vi "Main.vi"(10 "Module Admin":refnum<class "Delacor_lib_QMH_Module Admin.lvclass">, 11 "Sequence Context In":refnum<k7>) -> ()   [LabVIEW 2015, in "TestStand Manager_DQMH.lvlib"]
doc: "This application is based on the Delacor QMH project template. This particular module is headless, it has no UI, which is why the Show Panel, Hide Panel, and related events are unused.\n\nThe purpose of the TestStand Manager_DQMH Module is to check if the TestStand sequence is terminated. If so, it sends the request to stop all Thermal Chamber DQMH modules. This Module is only used when running the TestStand Examples.\n\n_____\nBased on Delacor QMH Project Template 2.0.0.62.\nReviewed and updated to match QMH Project Template 4.0.\n\n<b>Note:</b> This VI was modified by the <b>Validate DQMH Module</b> tool to upgrade it to the DQMH 2.1 approach to stopping a singleton module.\n\n<b>Note:</b> This VI was modified by the <b>Validate DQMH Module</b> tool to upgrade it to the DQMH 3.0 implementation of the 'Show Diagram' message, which checks the password-protected status of the Main VI before showing the diagram.\n____\nDelacor QMH Thermal Chamber Examples 4.0.0.21\nCopyright (c) 2018, Delacor"
uses:
  TestStand Manager_DQMH.lvlib
  Module Data--cluster.ctl
  <vilib>/Delacor/Delacor QMH/Libraries/Message Queue_class/Delacor_lib_QMH_Message Queue.lvclass
  <vilib>/Delacor/Delacor QMH/Libraries/Message Queue_class/Delacor_lib_QMH_Enqueue Message (Single).vi
  <vilib>/ErrorRing/Error Ring.xnode
  <vilib>/Utility/error.llb/Error Cluster From Error Code.vi
  <vilib>/Delacor/Delacor QMH/Libraries/Module Admin_class/Delacor_lib_QMH_Module Admin.lvclass
  Stop Argument--cluster.ctl
  <vilib>/addons/TestStand/_TSUtility.llb/TestStand - Status Monitor.ctl
  Thermal Chamber Controller_DQMH/Thermal Chamber Controller_DQMH.lvlib
  Device Under Test_Cloneable_DQMH/Device Under Test_Cloneable_DQMH.lvlib
panel:
  out "error out":errorcluster
  out "Status":string
  # "The purpose of the TestStand Manager_DQMH Module is to check if the TestStand sequence is terminated. If so, it sends the request to stop all Thermal Chamber DQMH modules. This Module is only used when running the TestStand Examples."
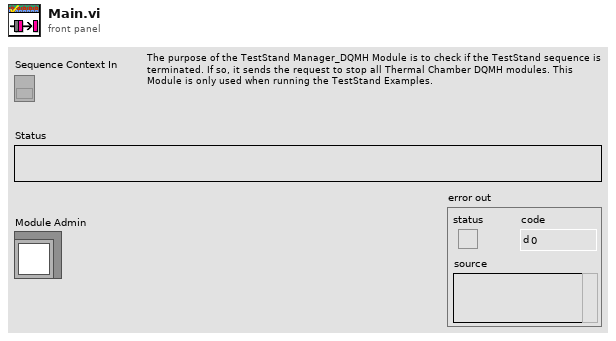
[diagram p1: front panel]
types:
  T1 = typedef "TestStand Manager_DQMH.lvlib/Request Events--cluster.ctl" = cluster{"Stop Module":refnum<user-event>, "Show Panel":refnum<user-event>, "Hide Panel":refnum<user-event>, "Get Module Execution Status":refnum<user-event>, "Show Diagram":refnum<user-event>}
  T2 = typedef "TestStand Manager_DQMH.lvlib/Module Data--cluster.ctl" = cluster{"Status":string, "Status Monitor":T3}
  T3 = typedef "TestStand - Status Monitor.ctl" = cluster{"Sequence Context":refnum<k7>, "Execution":refnum<k7>, "Termination Monitor":refnum<k7>}
  T4 = typedef "TestStand Manager_DQMH.lvlib/Stop Argument--cluster.ctl" = cluster{"Origin":string, "Exit via Stop Module Req?":bool, "Wait for Module to stop?":bool}
  T5 = enum32{"invalid lock state", "Not Locked", "Locked (No Password)", "Password-protected"}
  T6 = enum32{"Invalid", "Standard", "Closed", "Hidden", "Minimized", "Maximized"}
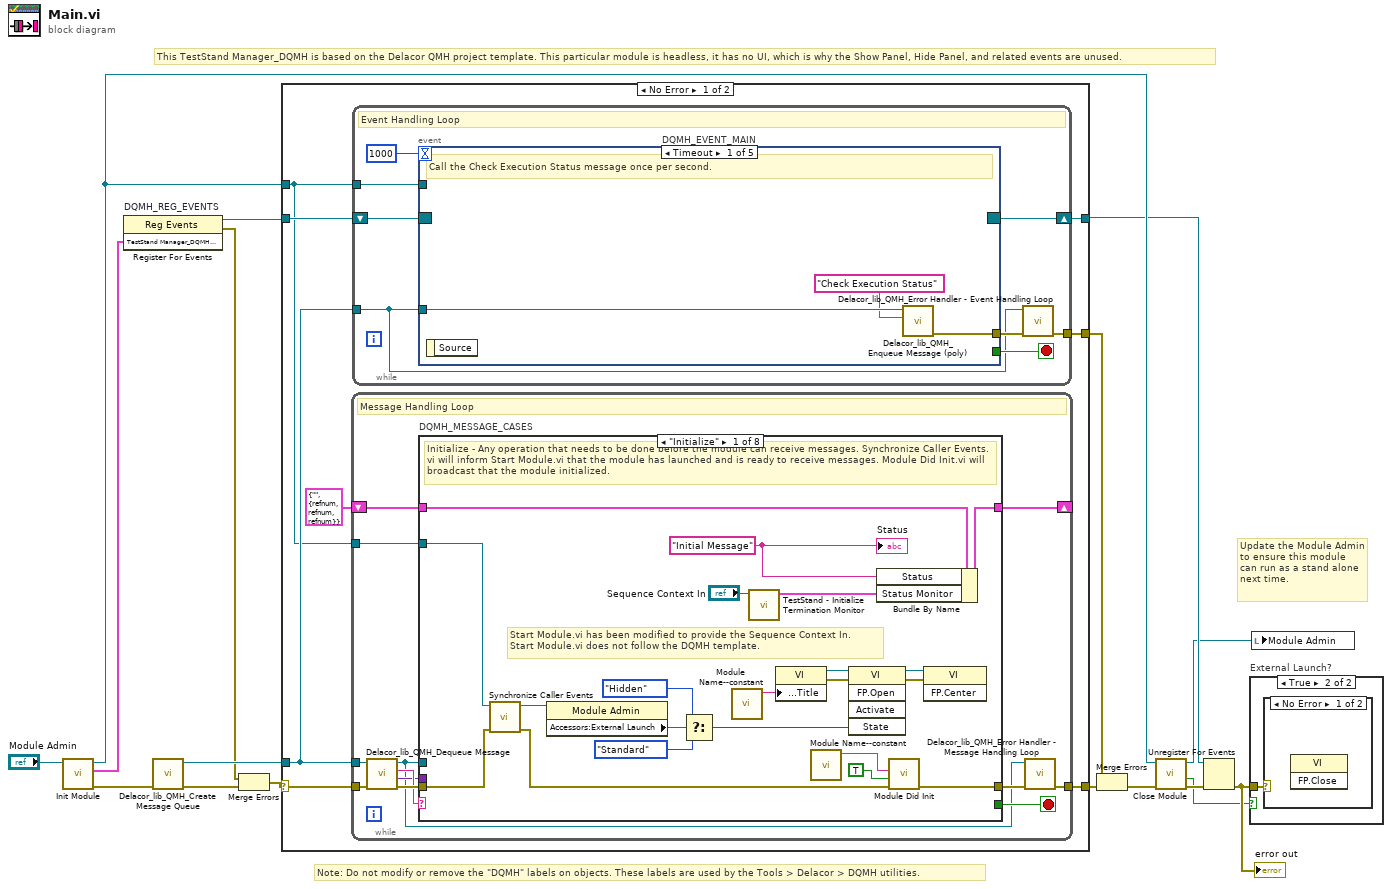
[diagram p0: block diagram]
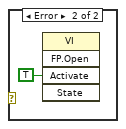
[diagram p3: hidden frame]
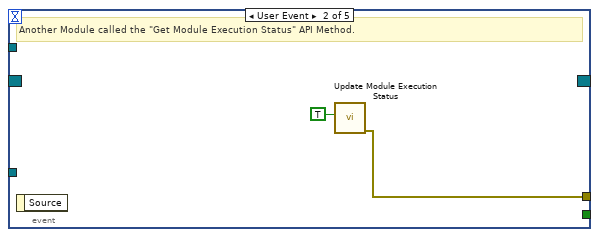
[diagram p4: hidden frame]
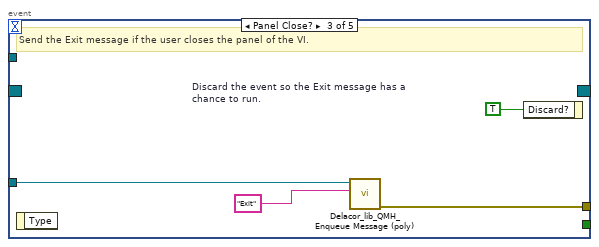
[diagram p5: hidden frame]
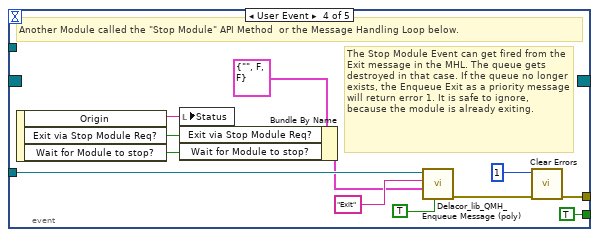
[diagram p6: hidden frame]
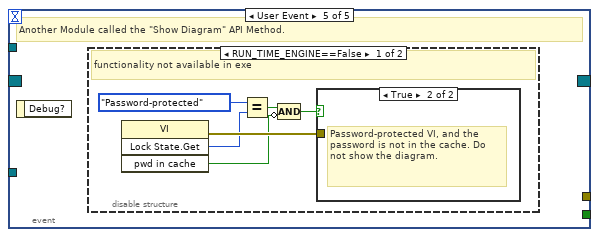
[diagram p7: hidden frame]
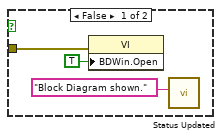
[diagram p8: hidden frame]
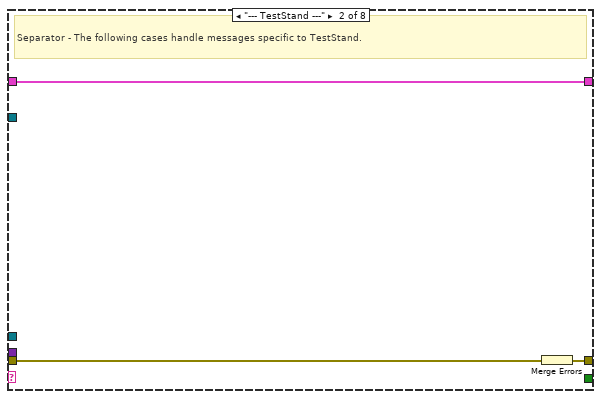
[diagram p10: hidden frame]
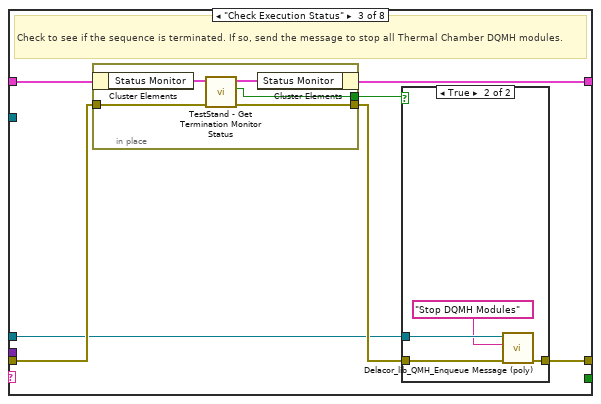
[diagram p11: hidden frame]
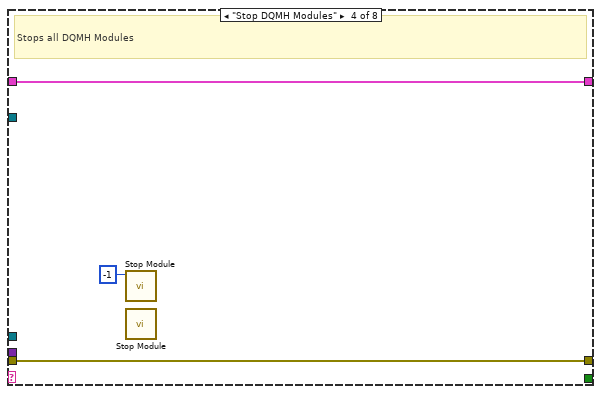
[diagram p13: hidden frame]
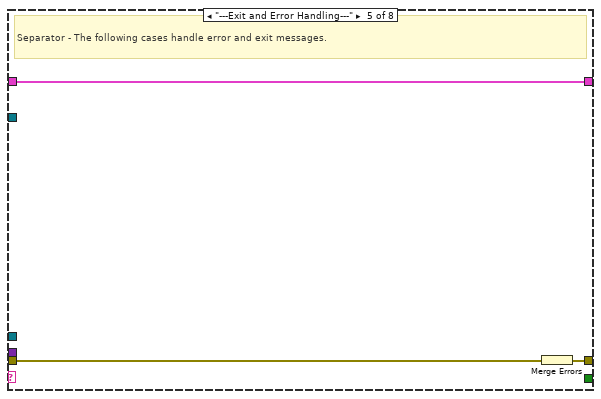
[diagram p14: hidden frame]
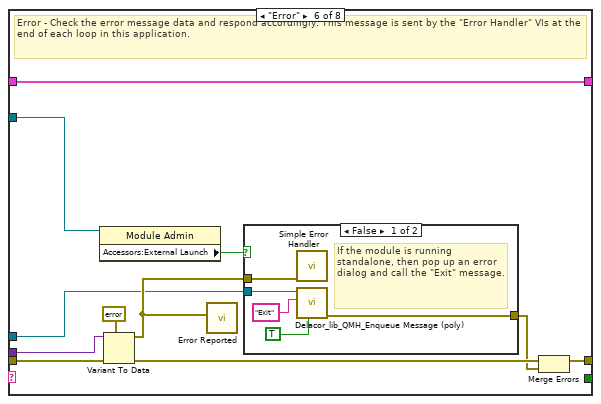
[diagram p15: hidden frame]
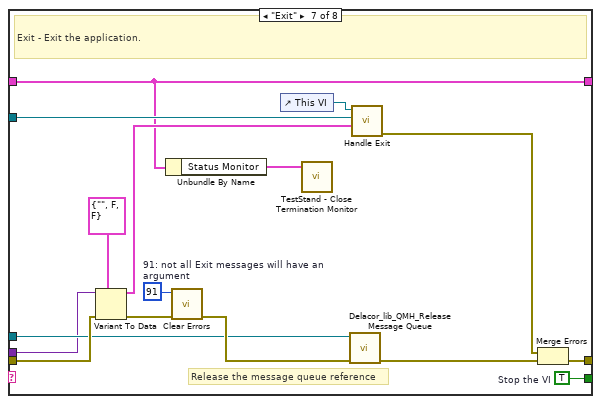
[diagram p17: hidden frame]
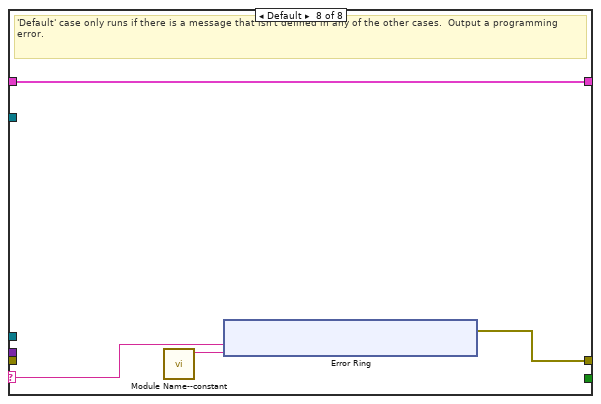
[diagram p18: hidden frame]
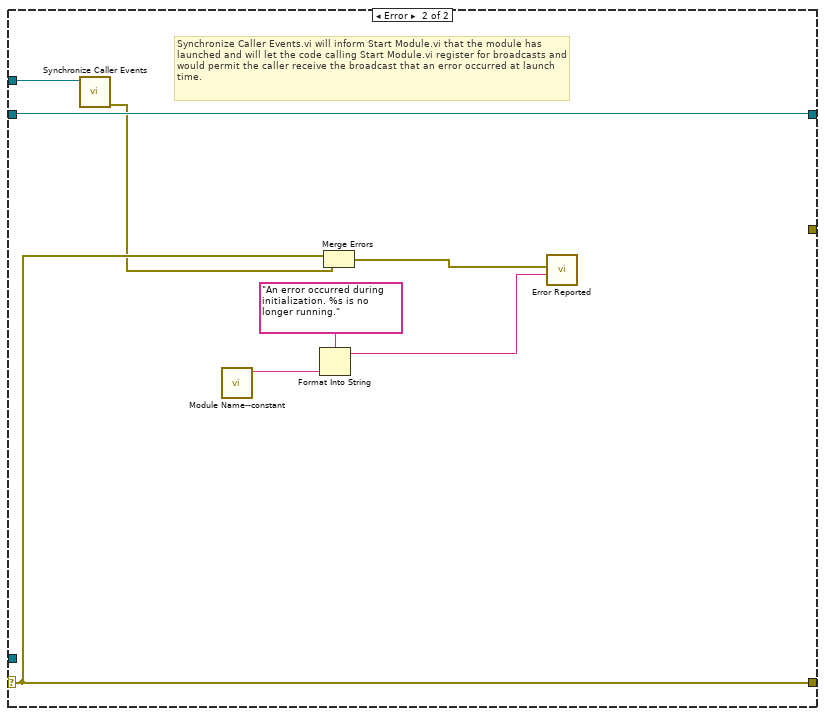
[diagram p19: hidden frame]
diagram:
  # "This TestStand Manager_DQMH is based on the Delacor QMH project template. This particular module is headless, it has no UI, which is why the Show Panel, Hide Panel, and related events are unused."
  # "Note: Do not modify or remove the \"DQMH\" labels on objects. These labels are used by the Tools > Delacor > DQMH utilities."
  # "Update the Module Admin to ensure this module can run as a stand alone next time."
  n1 = call "Init Module.vi"("Singleton Module Admin in"="Module Admin") -> ("error out"=w15:errorcluster, "TestStand Manager_DQMH Request Events"=w12:T1, "Singleton Module Admin out"=w17:refnum<class "Delacor_lib_QMH_Module Admin.lvclass">)  [unwired: 8 in]
  n2 = register-events "DQMH_REG_EVENTS"(w12) -> (reference out=w13:refnum<event-registration>, error out=w1:errorcluster)  [unwired: 2 in]
  n3 = call <vilib>:"Delacor_lib_QMH_Create Message Queue.vi"("error in (no error)"=w15) -> ("error out"=w3:errorcluster, "Message Queue out"=w11:refnum<class "Delacor_lib_QMH_Message Queue.lvclass">)  [unwired: 9 in]
  n4 = Merge Errors(w1, w3) -> (w2:errorcluster)
  n5 = case shown="No Error" w2 {
    selector: w2 -> [w19 w169]
    tunnel: [w25 w169] -> w16
    tunnel: [w24 w174] -> w14
    tunnel: w13 -> [w22 w174]
    tunnel: w11 -> [w21 _]
    tunnel: [w20 _] -> w7
    tunnel: w17 -> [w18 w170]
    frame No Error {
      n6 = while {
        tunnel: w21 -> [w67]
        shift-right: [w73] -> _
        shift-left: T2 {"Status"="", "Status Monitor"={"Sequence Context"=refnum, "Execution"=refnum, "Termination Monitor"=refnum}} ("Data Cluster") -> [w74]
        tunnel: w19 -> [w71]
        tunnel: [w65] -> w25
        tunnel: w18 -> [w64]
        stop <- w72 stop-if-true
        # "Message Handling Loop"
        n7 = call-dynamic "Delacor_lib_QMH_Dequeue Message.vi"("error in (no error)"=w71, "Message Queue in"=w67) -> ("error out"=w70:errorcluster, "Message Data"=w68:variant, "Message"=w69:string, "Message Queue out"=w66:refnum<class "Delacor_lib_QMH_Message Queue.lvclass">)  [unwired: 6 in]
        n8 = case "DQMH_MESSAGE_CASES" shown="\"Initialize\"" w69 {
          selector: w69 -> [_ _ _ _ _ _ _ w156]
          tunnel: w66 -> [_ _ w100 _ _ w125 w152 _]
          tunnel: w70 -> [w86 w99 w102 w117 w122 w132 w154 _]
          tunnel: [w80 w97 w101 w117 w120 w126 w149 w157] -> w75
          tunnel: w74 -> [w85 w98 w104 w119 w121 w131 w140 w158]
          tunnel: [w84 w98 w103 w119 w121 w131 w140 w158] -> w73
          tunnel: [_ _ _ _ _ _ w151 _] -> w72
          tunnel: w68 -> [_ _ _ _ _ w130 w148 _]
          tunnel: w64 -> [w87 _ _ _ _ w124 w141 _]
          frame "Initialize" {
            w76 = "Initial Message" ("Initial Message")
            # "Start Module.vi has been modified to provide the Sequence Context In.\nStart Module.vi does not follow the DQMH template."
            # "Initialize - Any operation that needs to be done before the module can receive messages. Synchronize Caller Events.vi will inform Start Module.vi that the module has launched and is ready to receive messages. Module Did Init.vi will broadcast that the module initialized."
            n9 = call "Synchronize Caller Events.vi"("error in (no error)"=w86, "Singleton Module Admin in"=w87) -> ("error out"=w81:errorcluster, "Singleton Module Admin out"=w79:refnum<class "Delacor_lib_QMH_Module Admin.lvclass">)  [unwired: 8 in]
            n10 = property on="Property Node" class="Module Admin"(reference=w79) -> ("Accessors:External Launch"=w91:bool)  [unwired: 1 in, 2 out]
            n11 = Select(t=T6."Hidden" ("State"), s=w91, f=T6."Standard" ("State")) -> (s? t:f=w88:T6)
            n12 = call "Module Name--constant.vi"() -> ("Module Name"=w96:string)  [unwired: 11 in]
            n13 = call <vilib>:"TestStand - Initialize Termination Monitor.vi"("Sequence Context In"="Sequence Context In") -> ("Status Monitor Out"=w77:T3)  [unwired: 9 in, 1 out]
            n14 = property on="Property Node" class="VI"("Front Panel.Title"=w96) -> (reference out=w94:refnum<vi>, error out=w95:errorcluster)  [unwired: 2 in]
            n15 = call "Module Name--constant.vi"() -> ("Module Name"=w82:string)  [unwired: 11 in]
            n16 = invoke on="Invoke Node" class="VI" method="FP.Open"(reference=w94, error in=w95, "State"=w88) -> (reference out=w93:refnum<vi>, error out=w92:errorcluster)  [unwired: 2 in, 3 out]
            n17 = Bundle By Name(cluster=w85, "Status"=w76, "Status Monitor"=w77) -> (w84:T2)
            n18 = call "Module Did Init.vi"("error in (no error)"=w81, "Initialized?"=TRUE, "Origin"=w82) -> ("error out"=w80:errorcluster)  [unwired: 8 in]
            n19 = invoke on="Invoke Node" class="VI" method="FP.Center"(reference=w93, error in=w92) -> ()  [unwired: 1 in, 3 out]
            "Status" <- w76
          }
          frame "--- TestStand ---" {
            # "Separator - The following cases handle messages specific to TestStand."
            n20 = Merge Errors(w99) -> (w97:errorcluster)
          }
          frame "Check Execution Status" {
            # "Check to see if the sequence is terminated. If so, send the message to stop all Thermal Chamber DQMH modules."
            n21 = in-place {
              in-place-border: w102 -> [w111]
              in-place-border: [w110] -> w106
              in-place-border: [w109] -> w105
              n22 = in-place-cluster #1(w104) -> ("Status Monitor"=w108:T3)
              n23 = call <vilib>:"TestStand - Get Termination Monitor Status.vi"("error in (no error)"=w111, "Status Monitor In"=w108) -> ("error out"=w110:errorcluster, "Terminating or Aborting"=w109:bool, "Status Monitor Out"=w107:T3)  [unwired: 7 in]
              n24 = in-place-cluster #1("Status Monitor"=w107) -> (w103:T2)
            }
            n25 = case shown="True" w105 {
              tunnel: w106 -> [w112 w116]
              tunnel: [w112 w115] -> w101
              tunnel: w100 -> [_ w114]
              frame False {
              }
              frame True {
                n26 = call-poly <vilib>:"Delacor_lib_QMH_Enqueue Message (poly).vi"("error in (no error)"=w116, "Message"="Stop DQMH Modules", "Message Queue in"=w114) -> ("error out"=w115:errorcluster)  [unwired: 7 in, 1 out]
              }
            }
          }
          frame "Stop DQMH Modules" {
            # "Stops all DQMH Modules"
            n27 = call "Stop Module.vi"("Module ID"=-1) -> ()  [unwired: 10 in, 1 out]
            n28 = call "Stop Module.vi"() -> ()  [unwired: 11 in, 1 out]
          }
          frame "---Exit and Error Handling---" {
            # "Separator - The following cases handle error and exit messages."
            n29 = Merge Errors(w122) -> (w120:errorcluster)
          }
          frame "Error" {
            # "Error - Check the error message data and respond accordingly. This message is sent by the \"Error Handler\" VIs at the end of each loop in this application."
            n30 = property on="Property Node" class="Module Admin"(reference=w124) -> ("Accessors:External Launch"=w123:bool)  [unwired: 1 in, 2 out]
            n31 = Variant To Data(error in=w132, type=errorcluster {"status"=FALSE, "code"=0, "source"=""} ("error constant"), Variant=w130) -> (data=w133:errorcluster, error out=w128:errorcluster)
            n32 = call "Error Reported.vi"("Error"=w133) -> ()  [unwired: 10 in, 1 out]
            n33 = case shown="False" w123 {
              tunnel: [w138 _] -> w127
              tunnel: w125 -> [w137 _]
              tunnel: w133 -> [w134 _]
              frame False {
                # "If the module is running standalone, then pop up an error dialog and call the \"Exit\" message."
                n34 = call <vilib>:"Simple Error Handler.vi"("error in (no error)"=w134) -> ()  [unwired: 4 in, 5 out]
                n35 = call-poly <vilib>:"Delacor_lib_QMH_Enqueue Message (poly).vi"("Priority Message? (F)"=TRUE, "Message"="Exit", "Message Queue in"=w137) -> ("error out"=w138:errorcluster)  [unwired: 7 in, 1 out]
              }
              frame True {
                # "If the module was launched externally, calling the Error Reported broadcast VI is the only action performed by the \"Error\" message. The module's caller can then process the error appropriately."
              }
            }
            n36 = Merge Errors(w128, w127) -> (w126:errorcluster)
          }
          frame "Exit" {
            w146 = 91  # 91: not all Exit messages will have an argument
            w151 = TRUE  # Stop the VI
            # "Release the message queue reference"
            # "Exit - Exit the application."
            n37 = Variant To Data(error in=w154, type=T4 {"Origin"="", "Exit via Stop Module Req?"=FALSE, "Wait for Module to stop?"=FALSE} ("Stop Argument"), Variant=w148) -> (data=w144:T4, error out=w147:errorcluster)
            n38 = Unbundle By Name(w140) -> ("Status Monitor"=w139:T3)
            n39 = call <vilib>:"Clear Errors.vi"("error in (no error)"=w147, "specific error code to clear (0: all)"=w146) -> ("error out"=w153:errorcluster)  [unwired: 4 in, 1 out]
            n40 = control-ref of="This VI"() -> (w142:refnum<vi>)
            n41 = call <vilib>:"TestStand - Close Termination Monitor.vi"("Status Monitor In"=w139) -> ()  [unwired: 10 in, 1 out]
            n42 = call-dynamic "Delacor_lib_QMH_Release Message Queue.vi"("error in (no error)"=w153, "Message Queue"=w152) -> ("error out"=w150:errorcluster)  [unwired: 9 in]
            n43 = call "Handle Exit.vi"("Stop Argument"=w144, "Admin in"=w141, "VI reference"=w142) -> ("error out"=w143:errorcluster)  [unwired: 7 in, 1 out]
            n44 = Merge Errors(w143, w150) -> (w149:errorcluster)
          }
          frame Default {
            # "'Default' case only runs if there is a message that isn't defined in any of the other cases.  Output a programming error."
            n45 = call "Module Name--constant.vi"() -> ("Module Name"=w155:string)  [unwired: 11 in]
            n46 = xnode "Error Ring"("parameter 0"=w156, "parameter 1"=w155) -> ("error out"=w157:errorcluster)
          }
        }
        n47 = call-dynamic "Delacor_lib_QMH_Error Handler - Message Handling Loop.vi"("error in (no error)"=w75, "Message Queue in"=w66) -> ("dup error in"=w65:errorcluster)  [unwired: 8 in, 1 out]
      }
      n48 = while {
        tunnel: w21 -> [w26]
        shift-right: [w32] -> w24
        shift-left: w22 -> [w33]
        tunnel: [w29] -> w20
        tunnel: w18 -> [w28]
        stop <- w30 stop-if-true
        # "Event Handling Loop"
        n49 = event "DQMH_EVENT_MAIN" shown="[0] Timeout" {
          selector: w33 -> [_ _ _ _ _]
          dyn-events: [_ _ _ _ _] -> w32
          timeout: 1000 -> [_ _ _ _ _]
          tunnel: [_ _ _ TRUE ("Discard?") _] -> w30
          tunnel: w26 -> [w36 _ w41 w52 _]
          tunnel: [w35 w38 w40 w47 _] -> w31
          tunnel: w28 -> [_ _ _ _ _]
          event Timeout {
            # "Call the Check Execution Status message once per second."
            n50 = event-data() -> ()  [unwired: 1 in, 1 out]
            n51 = call-poly <vilib>:"Delacor_lib_QMH_Enqueue Message (poly).vi"("Message"="Check Execution Status", "Message Queue in"=w36) -> ("error out"=w35:errorcluster)  [unwired: 8 in, 1 out]
          }
          event User Event {
            # "Another Module called the \"Get Module Execution Status\" API Method."
            n52 = event-data() -> ()  [unwired: 1 in, 1 out]
            n53 = call "Update Module Execution Status.vi"("Running?"=TRUE) -> ("error out"=w38:errorcluster)  [unwired: 10 in]
          }
          event Panel Close? {
            w42 = TRUE  # Discard the event so the Exit message has a chance to run.
            # "Send the Exit message if the user closes the panel of the VI."
            n54 = event-data() -> ()  [unwired: 1 in, 1 out]
            n55 = call-poly <vilib>:"Delacor_lib_QMH_Enqueue Message (poly).vi"("Message"="Exit", "Message Queue in"=w41) -> ("error out"=w40:errorcluster)  [unwired: 8 in, 1 out]
            n56 = event-data ("Event Filter Node")("Discard?"=w42) -> ()  [unwired: 1 in, 1 out]
          }
          event User Event {
            # "The Stop Module Event can get fired from the Exit message in the MHL. The queue gets destroyed in that case. If the queue no longer exists, the Enqueue Exit as a priority message will return error 1. It is safe to ignore, because the module is already exiting."
            # "Another Module called the \"Stop Module\" API Method  or the Message Handling Loop below."
            n57 = event-data() -> ("Origin"=w51:string, "Exit via Stop Module Req?"=w45:bool, "Wait for Module to stop?"=w44:bool)  [unwired: 1 in]
            n58 = local write "Status"(w51) -> ()
            n59 = Bundle By Name(cluster=T4 {"Origin"="", "Exit via Stop Module Req?"=FALSE, "Wait for Module to stop?"=FALSE} ("Stop Argument"), "Exit via Stop Module Req?"=w45, "Wait for Module to stop?"=w44) -> (w43:T4)
            n60 = call-poly <vilib>:"Delacor_lib_QMH_Enqueue Message (poly).vi"("Priority Message? (F)"=TRUE, "Message Data"=w43, "Message"="Exit", "Message Queue in"=w52) -> ("error out"=w48:errorcluster)  [unwired: 6 in, 1 out]
            n61 = call <vilib>:"Clear Errors.vi"("error in (no error)"=w48, "specific error code to clear (0: all)"=1) -> ("error out"=w47:errorcluster)  [unwired: 4 in, 1 out]
          }
          event User Event {
            # "Another Module called the \"Show Diagram\" API Method."
            n62 = event-data() -> ()  [unwired: 1 in, 1 out]
            n63 = disable-structure shown="RUN_TIME_ENGINE==False" {
              frame condition #0 (active) {
                # "functionality not available in exe"
                n64 = invoke on="Invoke Node" class="VI" method="Lock State.Get"() -> (error out=w60:errorcluster, "Get Lock State"=w59:T5, "pwd in cache"=w56:bool)  [unwired: 4 in, 1 out]
                n65 = Equal?(x=T5."Password-protected", y=w59) -> (x = y?=w57:bool)
                n66 = Compound Arithmetic op=AND(w57, invert w56) -> (w55:bool)
                n67 = case shown="True" w55 {
                  tunnel: w60 -> [w62 _]
                  frame False {
                    n68 = property on="Property Node" class="VI"(error in=w62, "BDWin.Open"=TRUE ("Block Diagram Window:Open")) -> ()  [unwired: 1 in, 2 out]
                    n69 = call "Status Updated.vi"("Status"="Block Diagram shown." ("format string")) -> ()  [unwired: 10 in, 1 out]
                  }
                  frame True {
                    # "Password-protected VI, and the password is not in the cache. Do not show the diagram."
                  }
                }
              }
              frame condition #1 {
              }
            }
          }
        }
        n70 = call-dynamic "Delacor_lib_QMH_Error Handler - Event Handling Loop.vi"("error in (no error)"=w31, "Message Queue in"=w26) -> ("dup error in"=w29:errorcluster)  [unwired: 8 in, 1 out]
      }
    }
    frame Error {
      # "Synchronize Caller Events.vi will inform Start Module.vi that the module has launched and will let the code calling Start Module.vi register for broadcasts and would permit the caller receive the broadcast that an error occurred at launch time."
      n71 = call "Synchronize Caller Events.vi"("Singleton Module Admin in"=w170) -> ("error out"=w167:errorcluster)  [unwired: 9 in, 1 out]
      n72 = call "Module Name--constant.vi"() -> ("Module Name"=w173:string)  [unwired: 11 in]
      n73 = Format Into String(format string="An error occurred during initialization. %s is no longer running.", w173) -> (resulting string=w171:string)  [unwired: 2 in, 1 out]
      n74 = Merge Errors(w169, w167) -> (w168:errorcluster)
      n75 = call "Error Reported.vi"("Additional Information"=w171, "Error"=w168) -> ()  [unwired: 9 in, 1 out]
    }
  }
  n76 = Merge Errors(w7, w16) -> (w6:errorcluster)
  n77 = call "Close Module.vi"("error in (no error)"=w6, "Module Admin in"=w17) -> ("error out"=w9:errorcluster, "External Launch"=w4:bool, "Module Admin out"=w8:refnum<class "Delacor_lib_QMH_Module Admin.lvclass">)  [unwired: 7 in]
  n78 = Unregister For Events(event registration refnum=w14, error in=w9) -> (error out=w5:errorcluster)
  "error out" <- w5
  n79 = case "External Launch?" shown="True" w4 {
    tunnel: w5 -> [_ w175]
    frame False {
    }
    frame True {
      n80 = case shown="No Error" w175 {
        frame No Error {
          n81 = invoke on="Invoke Node" class="VI" method="FP.Close"() -> ()  [unwired: 3 in, 3 out]
        }
        frame Error {
          n82 = invoke on="Invoke Node" class="VI" method="FP.Open"("Activate"=TRUE ("Activate?")) -> ()  [unwired: 4 in, 5 out]
        }
      }
    }
  }
  n83 = local write "Module Admin"(w8) -> ()
